vi "Destructor.vi"(8 "error in":errorcluster, 11 "Datawarehouse":refnum<class "Datawarehouse.lvclass">) -> (0 "error out":errorcluster)   [LabVIEW 2021, in "ProligentXMLGenerator.lvlib" / "Datawarehouse.lvclass"]
doc: "Closes the ProligentCanonicalFile in memory"
uses:
  Datawarehouse.lvclass
  Datawarehouse.lvclass/Datawarehouse.ctl
  Failure/Defect/Defect.lvclass
  <vilib>/xml/NI_XML.lvlib
  ProcessRun/ProcessRun.lvclass
  <vilib>/xml/Close Reference(Node).vi
  ProductUnit/ProductUnit.lvclass
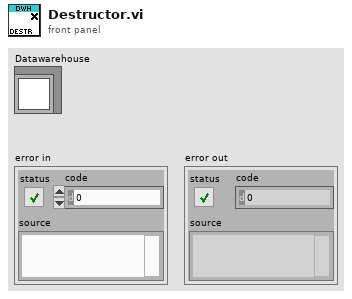
[diagram p1: front panel]
types:
  T1 = typedef "ProligentXMLGenerator.lvlib/Datawarehouse.lvclass/Data.ctl" = cluster{"DestinationFolder":path, "BaseFileName":string, "Document":refnum<k20>, "Defects":refnum<class "Defect.lvclass">[], "TopProcessRuns":refnum<class "ProcessRun.lvclass">[], "ProductUnits":refnum<class "ProductUnit.lvclass">[], "GenerationTime":refnum<class "DateTime.lvclass">, "DataSourceFingerprint":refnum<class "NonEmptyString_448.lvclass">, "IntegrationMetaData":refnum<class "NonEmptyString_2000.lvclass">, "TimeZoneInfoId":string}
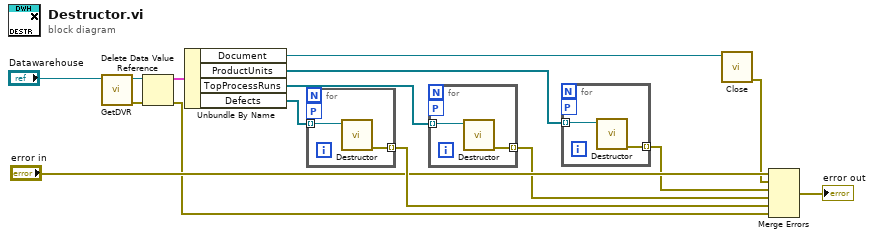
[diagram p0: block diagram]
diagram:
  n1 = call "GetDVR.vi"("Datawarehouse"="Datawarehouse") -> ("error out"=w7:errorcluster, "DVRReference"=w8:refnum<data-value>)  [unwired: 9 in]
  n2 = Delete Data Value Reference(data value reference=w8, error in=w7) -> (data value=w6:T1, error out=w3:errorcluster)
  n3 = Unbundle By Name(w6) -> ("Document"=w11:refnum<k20>, "ProductUnits"=w1:refnum<class "ProductUnit.lvclass">[], "TopProcessRuns"=w4:refnum<class "ProcessRun.lvclass">[], "Defects"=w12:refnum<class "Defect.lvclass">[])
  n4 = for {
    tunnel: w12 -> [w17] mode=indexing
    tunnel: [w16] -> w15 mode=indexing
    workers-P: _ -> [_]
    n5 = call "Destructor.vi"("Defect"=w17) -> ("error out"=w16:errorcluster)  [unwired: 10 in]
  }
  n6 = for {
    tunnel: w4 -> [w19] mode=indexing
    tunnel: [w18] -> w5 mode=indexing
    workers-P: _ -> [_]
    n7 = call "Destructor.vi"("ProcessRun in"=w19) -> ("error out"=w18:errorcluster)  [unwired: 10 in]
  }
  n8 = for {
    tunnel: w1 -> [w21] mode=indexing
    tunnel: [w20] -> w2 mode=indexing
    workers-P: _ -> [_]
    n9 = call "Destructor.vi"("ProductUnit in"=w21) -> ("error out"=w20:errorcluster)  [unwired: 10 in]
  }
  n10 = call-poly <vilib>:"Close.vi"("node"=w11) -> ("error out"=w10:errorcluster)  [unwired: 8 in]
  n11 = Merge Errors("error in", w10, w2, w5, w15, w3) -> (→"error out":errorcluster)
